vi "Send Single TCP-IP Cmd 1.vi"(0 "TCP/IP ID":refnum<k5>, 1 "Buffer/Avg #/Frames":u16, 2 "Mode":u16, 3 "Exposure Time (ms)":u32, 4 "Camera Color":string(combo), 5 "Error In":errorcluster, 6 "Function #":u16, 7 "File Name":string, 9 "Parameter Value":i32, 10 "Camera ID":u8=1, 11 "Save As":u16(ring) items=["U16 FITS", "I16 FITS", "I32 FITS", "SGL FITS", "U16 TIFF", "I16 TIFF", "I32 TIFF", "SGL TIFF"], 12 "Acq. Mode/Type/Frame Mode/RO Mode #":u8, 13 "CCD Format Parameters":T1={"Serial Origin"=50, "Serial Length"=512, "Serial Binning"=1, "Parallel Origin"=0, "Parallel Length"=1024, "Parallel Binning"=1} {"Parallel Binning" min=1 max=5000 step=1; "Parallel Length" min=0 max=65535 step=1; "Parallel Origin" min=0 max=9000 step=1; "Serial Binning" min=1 max=5000 step=1; "Serial Length" min=0 max=65535 step=1; "Serial Origin" min=0 max=9000 step=1}) -> (14 "TCP/IP ID Out":refnum<k5>, 15 "Cmd Packet":string, 17 "Read String":string, 19 "Error Out":errorcluster)   [LabVIEW 2015]
uses:
  CCD Format.ctl
panel:
  # "Parallel"
  # "Serial"
  # "Origin"
  # "Length"
  # "Binning"
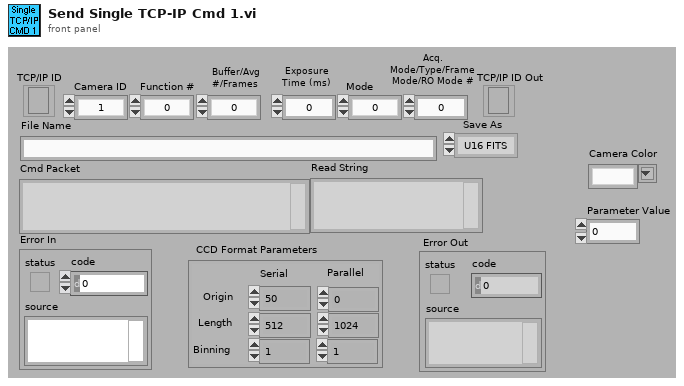
[diagram p1: front panel]
types:
  T1 = typedef "CCD Format.ctl" = cluster{"Serial Origin":i32, "Serial Length":i32, "Serial Binning":i32, "Parallel Origin":i32, "Parallel Length":i32, "Parallel Binning":i32}
  T2 = cluster{"% Exp.":u16, "%Readout":u16, "Relative Pos.":u32, "Acquiring":i32}
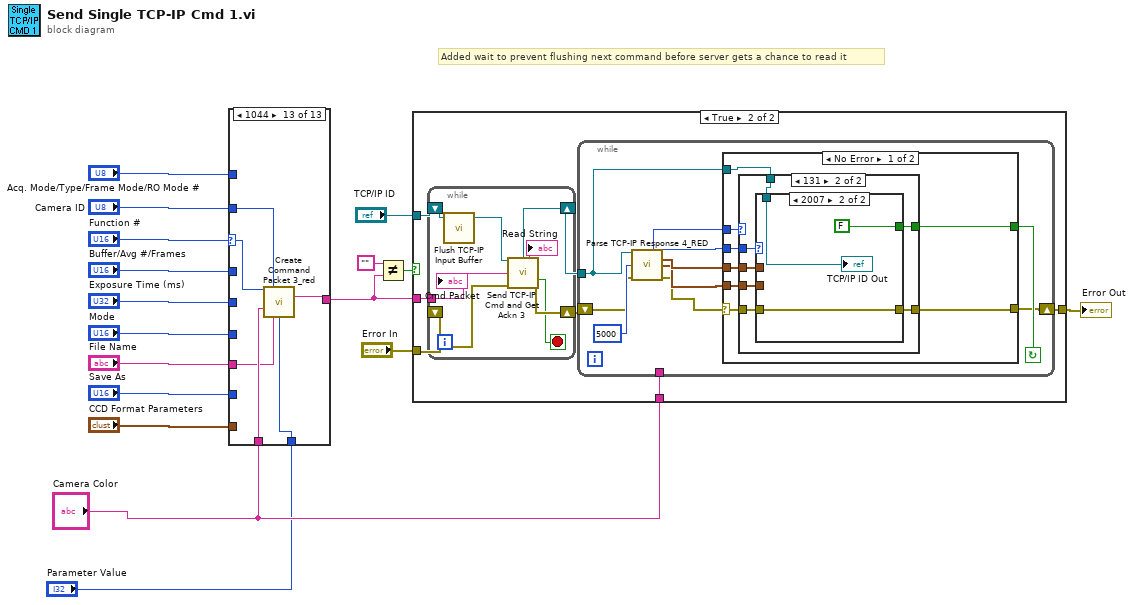
[diagram p0: block diagram]
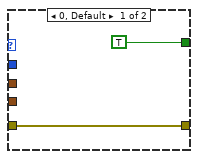
[diagram p3: hidden frame]
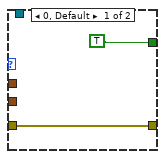
[diagram p4: hidden frame]
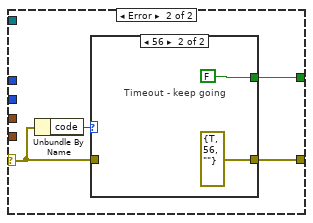
[diagram p5: hidden frame]
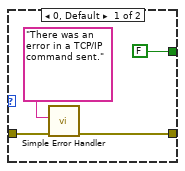
[diagram p6: hidden frame]
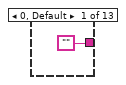
[diagram p7: hidden frame]
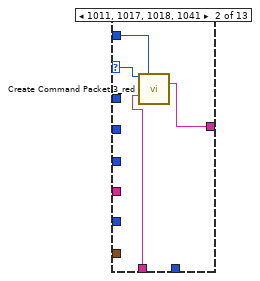
[diagram p8: hidden frame]
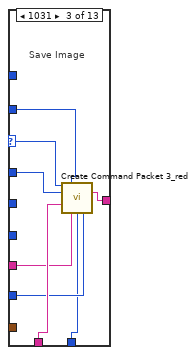
[diagram p9: hidden frame]
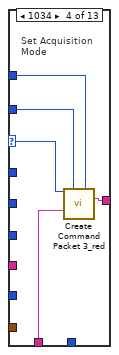
[diagram p10: hidden frame]
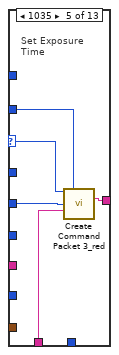
[diagram p11: hidden frame]
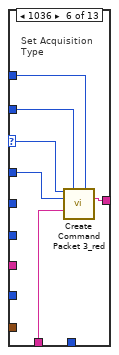
[diagram p12: hidden frame]
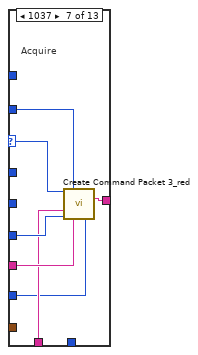
[diagram p13: hidden frame]
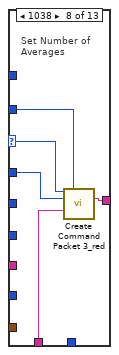
[diagram p14: hidden frame]
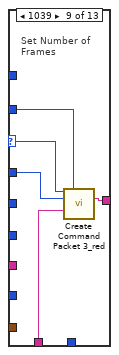
[diagram p15: hidden frame]
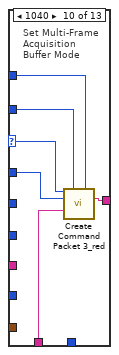
[diagram p16: hidden frame]
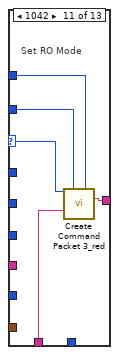
[diagram p17: hidden frame]
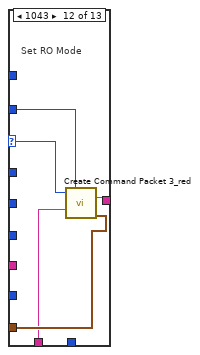
[diagram p18: hidden frame]
diagram:
  # "Added wait to prevent flushing next command before server gets a chance to read it"
  n1 = case shown="1044" "Function #" {
    selector: "Function #" -> [_ w20 w28 w33 w38 w44 w51 w56 w61 w67 w72 w78 w80]
    tunnel: ["" w22 w24 w35 w40 w46 w53 w58 w63 w69 w74 w79 w85] -> w8
    tunnel: "Acq. Mode/Type/Frame Mode/RO Mode #" -> [_ _ _ w32 _ w43 _ _ _ w65 w71 _ _]
    tunnel: "Camera ID" -> [_ w21 w29 w34 w39 w45 w52 w57 w62 w68 w73 w77 w81]
    tunnel: "Buffer/Avg #/Frames" -> [_ _ w27 _ _ w42 _ w55 w60 w66 _ _ _]
    tunnel: "Exposure Time (ms)" -> [_ _ _ _ w37 _ _ _ _ _ _ _ _]
    tunnel: "Mode" -> [_ _ _ _ _ _ w49 _ _ _ _ _ _]
    tunnel: "File Name" -> [_ _ w26 _ _ _ w50 _ _ _ _ _ w82]
    tunnel: "Save As" -> [_ _ w25 _ _ _ w47 _ _ _ _ _ _]
    tunnel: "CCD Format Parameters" -> [_ _ _ _ _ _ _ _ _ _ _ w76 _]
    tunnel: "Camera Color" -> [_ w19 w30 w31 w36 w41 w48 w54 w59 w64 w70 w75 w84]
    tunnel: "Parameter Value" -> [_ _ w23 _ _ _ _ _ _ _ _ _ w83]
    frame 0, Default {
    }
    frame 1011, 1017, 1018, 1041 {
      n2 = call "Create Command Packet 3_red.vi"("Function #"=w20, "Camera ID (1)"=w21, "Camera Color"=w19) -> ("Cmd Packet"=w22:string)  [unwired: 12 in]
    }
    frame 1031 {
      # "Save Image"
      n3 = call "Create Command Packet 3_red.vi"("Function #"=w28, "Camera ID (1)"=w29, "Buffer/Avg #/Frames"=w27, "Camera Color"=w30, "File Name"=w26, "Paramater value"=w23, "Save As"=w25) -> ("Cmd Packet"=w24:string)  [unwired: 8 in]
    }
    frame 1034 {
      # "Set Acquisition Mode"
      n4 = call "Create Command Packet 3_red.vi"("Function #"=w33, "Camera ID (1)"=w34, "Acq. Mode/Type/Frame Mode/RO Mode"=w32, "Camera Color"=w31) -> ("Cmd Packet"=w35:string)  [unwired: 11 in]
    }
    frame 1035 {
      # "Set Exposure Time"
      n5 = call "Create Command Packet 3_red.vi"("Function #"=w38, "Camera ID (1)"=w39, "Exposure Time (ms)"=w37, "Camera Color"=w36) -> ("Cmd Packet"=w40:string)  [unwired: 11 in]
    }
    frame 1036 {
      # "Set Acquisition Type"
      n6 = call "Create Command Packet 3_red.vi"("Function #"=w44, "Camera ID (1)"=w45, "Acq. Mode/Type/Frame Mode/RO Mode"=w43, "Buffer/Avg #/Frames"=w42, "Camera Color"=w41) -> ("Cmd Packet"=w46:string)  [unwired: 10 in]
    }
    frame 1037 {
      # "Acquire"
      n7 = call "Create Command Packet 3_red.vi"("Function #"=w51, "Camera ID (1)"=w52, "Camera Color"=w48, "Mode"=w49, "File Name"=w50, "Save As"=w47) -> ("Cmd Packet"=w53:string)  [unwired: 9 in]
    }
    frame 1038 {
      # "Set Number of Averages"
      n8 = call "Create Command Packet 3_red.vi"("Function #"=w56, "Camera ID (1)"=w57, "Buffer/Avg #/Frames"=w55, "Camera Color"=w54) -> ("Cmd Packet"=w58:string)  [unwired: 11 in]
    }
    frame 1039 {
      # "Set Number of Frames"
      n9 = call "Create Command Packet 3_red.vi"("Function #"=w61, "Camera ID (1)"=w62, "Buffer/Avg #/Frames"=w60, "Camera Color"=w59) -> ("Cmd Packet"=w63:string)  [unwired: 11 in]
    }
    frame 1040 {
      # "Set Multi-Frame Acquisition Buffer Mode"
      n10 = call "Create Command Packet 3_red.vi"("Function #"=w67, "Camera ID (1)"=w68, "Acq. Mode/Type/Frame Mode/RO Mode"=w65, "Buffer/Avg #/Frames"=w66, "Camera Color"=w64) -> ("Cmd Packet"=w69:string)  [unwired: 10 in]
    }
    frame 1042 {
      # "Set RO Mode"
      n11 = call "Create Command Packet 3_red.vi"("Function #"=w72, "Camera ID (1)"=w73, "Acq. Mode/Type/Frame Mode/RO Mode"=w71, "Camera Color"=w70) -> ("Cmd Packet"=w74:string)  [unwired: 11 in]
    }
    frame 1043 {
      # "Set RO Mode"
      n12 = call "Create Command Packet 3_red.vi"("Function #"=w78, "Camera ID (1)"=w77, "Camera Color"=w75, "CCD Format Parameters"=w76) -> ("Cmd Packet"=w79:string)  [unwired: 11 in]
    }
    frame 1044 {
      n13 = call "Create Command Packet 3_red.vi"("Function #"=w80, "Camera ID (1)"=w81, "Camera Color"=w84, "File Name"=w82, "Paramater value"=w83) -> ("Cmd Packet"=w85:string)  [unwired: 10 in]
    }
  }
  n14 = Not Equal?(x="", y=w8) -> (x != y?=w9:bool)
  n15 = case shown="True" w9 {
    tunnel: w8 -> [_ w93]
    tunnel: "TCP/IP ID" -> [_ w91]
    tunnel: "Error In" -> [w86 w90]
    tunnel: [w86 w89] -> w5
    tunnel: "Camera Color" -> [_ w88]
    frame False {
    }
    frame True {
      n16 = while {
        tunnel: w93 -> [w99]
        shift-right: [w98] -> w92
        shift-left: w91 -> [w97]
        shift-right: [w95] -> w87
        shift-left: w90 -> [w96]
        stop <- w94 stop-if-true
        n17 = call "Flush TCP-IP Input Buffer.vi"("TCP/IP ID"=w97) -> ("TCP/IP ID Out"=w100:refnum<k5>)  [unwired: 4 in]
        n18 = call "Send TCP-IP Cmd and Get Ackn 3.vi"("TCP/IP ID In"=w100, "Cmd Packet"=w99, "error in (no error)"=w96) -> ("TCP/IP ID Out"=w98:refnum<k5>, "Read String"=→"Read String":string, "Accepted Flag"=w94:bool, "error out"=w95:errorcluster)  [unwired: 6 in, 3 out]
        "Cmd Packet" <- w99
      }
      n19 = while {
        tunnel: w92 -> [w104]
        shift-right: [w106] -> w89
        shift-left: w87 -> [w102]
        tunnel: w88 -> [_]
        stop <- w107 continue-if-true
        n20 = call "Parse TCP-IP Response 4_RED.vi"("TCP/IP ID"=w104, "timeout ms (5000)"=5000, "error in (no error)"=w102) -> ("Packet ID"=w105:u8, "Data Type"=w108:u16, "Command Done"=w111:cluster{"Function #":u16}, "Acq. Status"=w110:T2, "error out"=w109:errorcluster)  [unwired: 2 in, 6 out]
        n21 = case shown="No Error" w109 {
          selector: w109 -> [w114 w135]
          tunnel: w105 -> [w119 _]
          tunnel: w111 -> [w118 _]
          tunnel: w110 -> [w117 _]
          tunnel: [w116 w137] -> w107
          tunnel: w108 -> [w115 _]
          tunnel: [w113 w134] -> w106
          tunnel: w104 -> [w112 _]
          frame No Error {
            n22 = case shown="131" w119 {
              tunnel: w118 -> [_ w123]
              tunnel: w117 -> [_ w128]
              tunnel: [TRUE w127] -> w116
              tunnel: w115 -> [_ w126]
              tunnel: w114 -> [w120 w125]
              tunnel: [w120 w124] -> w113
              tunnel: w112 -> [_ w122]
              frame 0, Default {
              }
              frame 131 {
                n23 = case shown="2007" w126 {
                  tunnel: w128 -> [_ _]
                  tunnel: [TRUE FALSE] -> w127
                  tunnel: [w129 w132] -> w124
                  tunnel: w125 -> [w129 w132]
                  tunnel: w123 -> [_ _]
                  tunnel: w122 -> [_ w131]
                  frame 0, Default {
                  }
                  frame 2007 {
                    "TCP/IP ID Out" <- w131
                  }
                }
              }
            }
          }
          frame Error {
            n24 = Unbundle By Name(w135) -> ("code"=w136:i32)
            n25 = case shown="56" w136 {
              tunnel: w135 -> [w141 _]
              tunnel: [FALSE FALSE] -> w137
              tunnel: [w138 errorcluster {"status"=TRUE, "code"=56, "source"=""} ("error out")] -> w134
              frame 0, Default {
                n26 = call <vilib>:"Simple Error Handler.vi"("error source (\" \")"="There was an error in a TCP/IP command sent.", "error in (no error)"=w141) -> ("error out"=w138:errorcluster)  [unwired: 3 in, 4 out]
              }
              frame 56 {
                # "Timeout - keep going"
              }
            }
          }
        }
      }
    }
  }
  "Error Out" <- w5
